vi "Row size.vi"() -> ()   [LabVIEW 2022 SP3]
panel:
  out "row size":i32
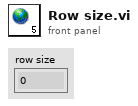
[diagram p1: front panel]
diagram:
